vi "ZZZZZZZZ.vi"(7 "Actor":refnum<class "Actor Layer.lvclass">, 11 "Actor":T1) -> (3 "Actor":T1, 4 "Error":errorcluster, 5 "Actor":refnum<class "Actor Layer.lvclass">)   [LabVIEW 2020, in "jettl.lvlib"]
uses:
  jettl.lvlib
  Lifecycle.ctl
  Actor Layer/Actor Layer.lvclass
  Msg/Msg.lvclass
  Origin.ctl
  Msg Attribs.ctl
  Msg.ctl
  Post Setup.ctl
  Pre Setup.ctl
  Msg Set.ctl
  Actor Attribs.ctl
  Children.ctl
  Actor.ctl
  Layer Type.ctl
  Layer Attribs.ctl
  Layer Map.ctl
  Implemented Map.ctl
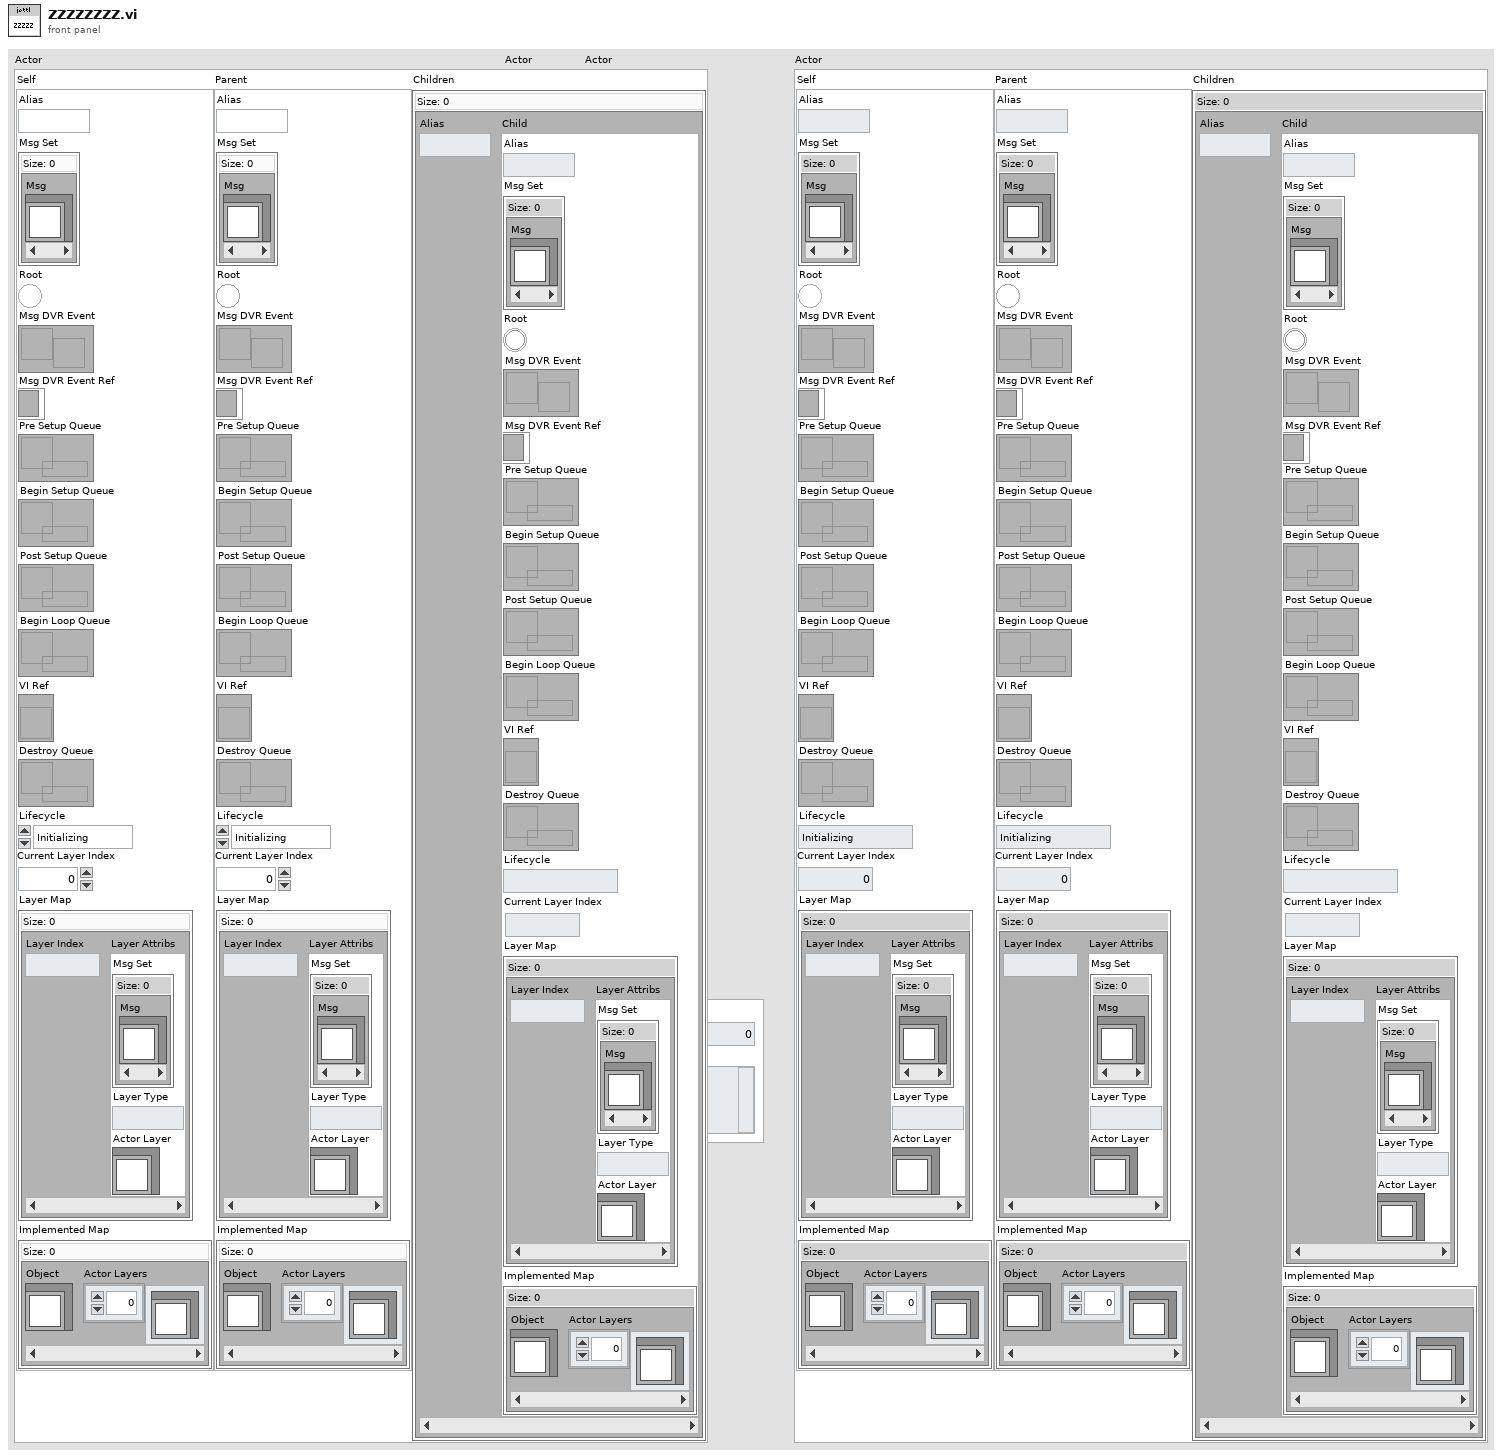
[diagram p1: front panel]
types:
  T1 = typedef "jettl.lvlib/Actor.ctl" = cluster{"Self":T2, "Parent":T2, "Children":T9}
  T2 = typedef "jettl.lvlib/Actor Attribs.ctl" = cluster{"Alias":string, "Msg Set":T3, "Root":bool, "Msg DVR Event":refnum<user-event>, "Msg DVR Event Ref":refnum<event-registration>, "Pre Setup Queue":refnum<queue>, "Begin Setup Queue":refnum<queue>, "Post Setup Queue":refnum<queue>, "Begin Loop Queue":refnum<queue>, "VI Ref":refnum<vi>, "Destroy Queue":refnum<queue>, "Lifecycle":T4, "Current Layer Index":i32, "Layer Map":T5, "Implemented Map":T8}
  T3 = typedef "jettl.lvlib/Msg Set.ctl" = set{refnum<class "Msg.lvclass">}
  T4 = typedef "jettl.lvlib/Lifecycle.ctl" = enum16{"Initializing", "Setting Up", "Starting", "Running", "Stopping", "Tearing Down", "Terminated"}
  T5 = typedef "jettl.lvlib/Layer Map.ctl" = map{i32, T6}
  T6 = typedef "jettl.lvlib/Layer Attribs.ctl" = cluster{"Msg Set":T3, "Layer Type":T7, "Actor Layer":refnum<class "Actor Layer.lvclass">}
  T7 = typedef "jettl.lvlib/Layer Type.ctl" = enum16{"Base", "InnerGlobal", "InnerLocal", "Outer"}
  T8 = typedef "jettl.lvlib/Implemented Map.ctl" = map{refnum<class>, refnum<class "Actor Layer.lvclass">[]}
  T9 = typedef "jettl.lvlib/Children.ctl" = map{string, T2}
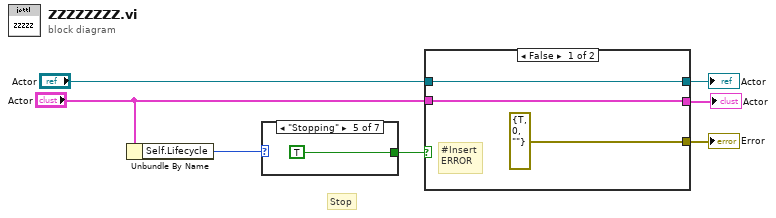
[diagram p0: block diagram]
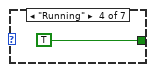
[diagram p5: hidden frame]
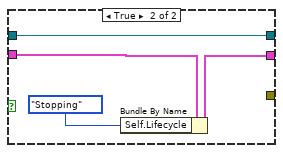
[diagram p8: hidden frame]
diagram:
  # "Stop"
  n1 = Unbundle By Name("Actor") -> ("Self.Lifecycle"=w5:T4)
  n2 = case shown="\"Stopping\"" w5 {
    tunnel: [_ _ _ TRUE TRUE _ _] -> w4
    frame "Initializing" {
    }
    frame "Setting Up" {
    }
    frame "Starting" {
    }
    frame "Running" {
    }
    frame "Stopping" {
    }
    frame "Tearing Down" {
    }
    frame "Terminated" {
    }
  }
  n3 = case shown="False" w4 {
    tunnel: [w12 w16] -> w7
    tunnel: "Actor" -> [w12 w16]
    tunnel: [errorcluster {"status"=TRUE, "code"=0, "source"=""} ("Error") _] -> w3
    tunnel: [w10 w14] -> w2
    tunnel: "Actor" -> [w10 w13]
    frame False {
      # "#Insert\nERROR"
    }
    frame True {
      n4 = Bundle By Name(cluster=w13, "Self.Lifecycle"=Lifecycle."Stopping" ("Lifecycle")) -> (w14:T1)
    }
  }
  "Actor" <- w7
  "Error" <- w3
  "Actor" <- w2
